vi "Simple Line Detection Control System.vi"() -> ()   [LabVIEW 2017]
panel:
  out "?":string
  in  "Right Sensor":bool=TRUE
  in  "Middle Sensor":bool
  in  "Left Sensor":bool=TRUE
  in  "Stop":bool
  out "Direction":string
  out "Speedometer (m/s)":dbl(knob) scale=0.0..3.0
  in  "% Power":dbl(slide) scale=0.0..100.0
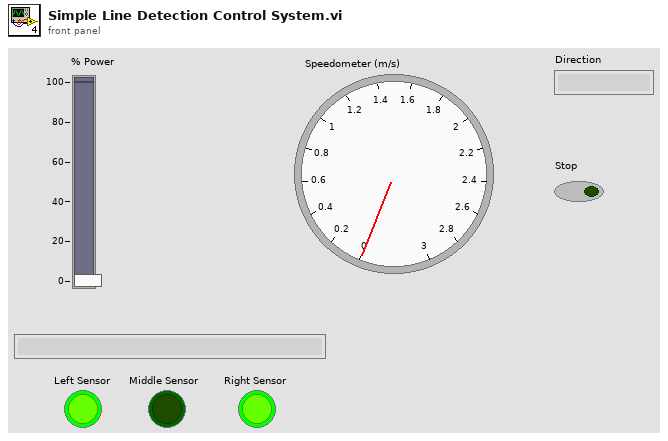
[diagram p1: front panel]
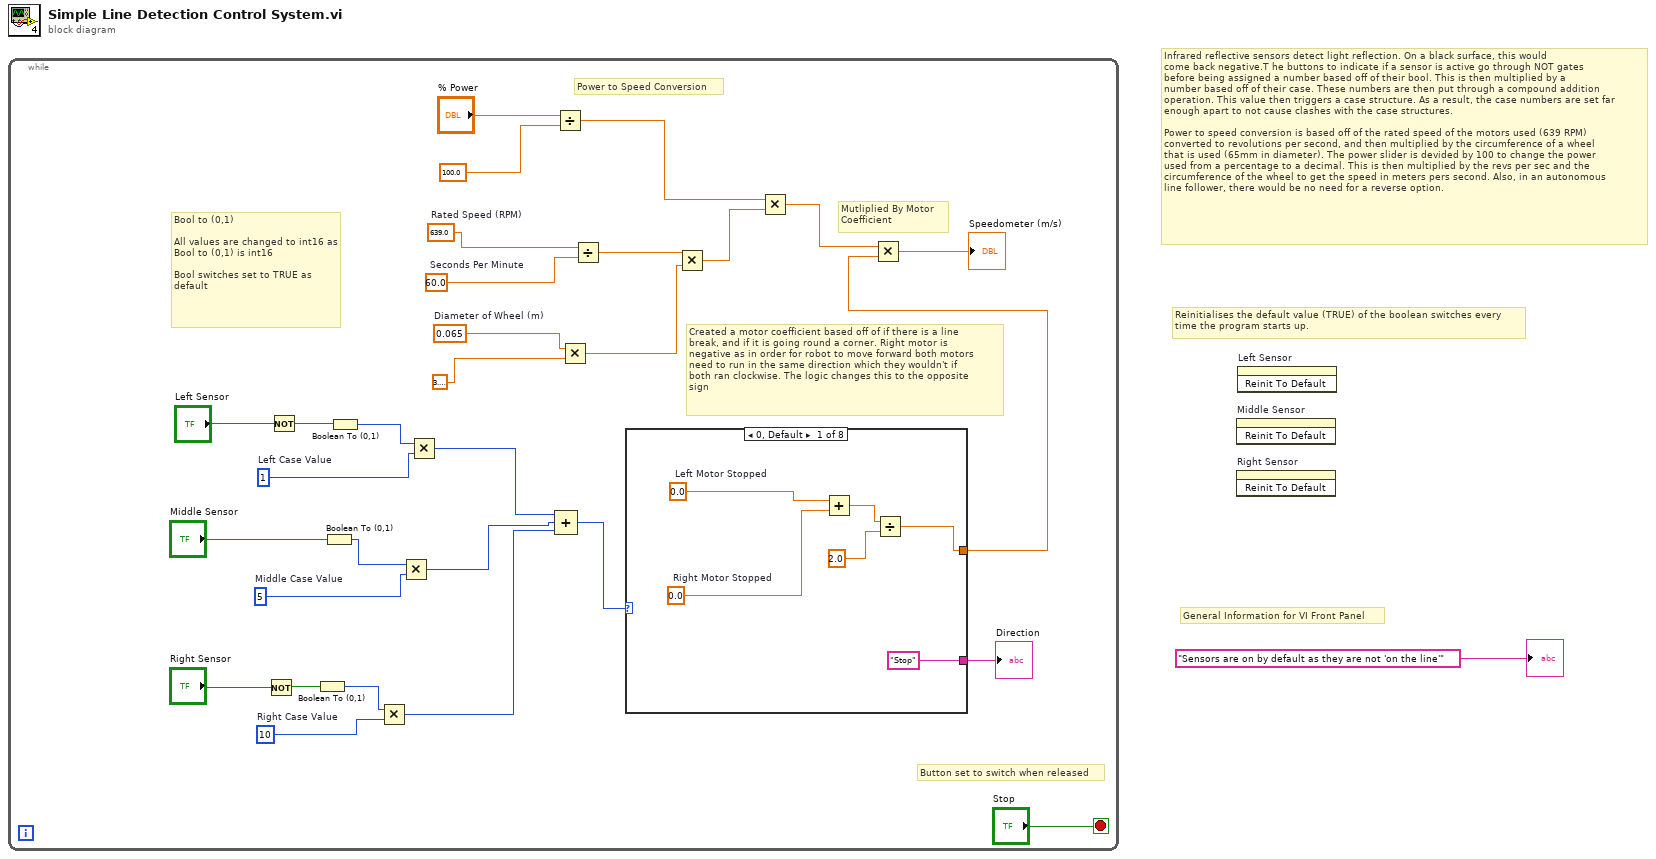
[diagram p0: block diagram]
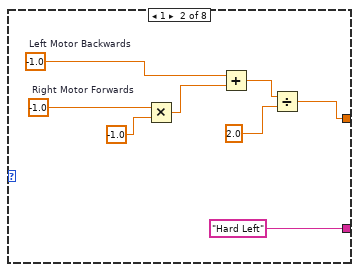
[diagram p2: hidden frame]
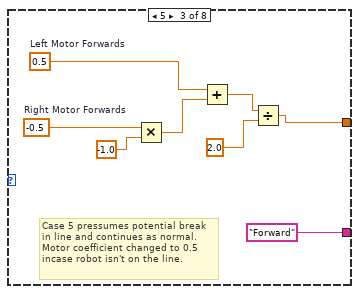
[diagram p3: hidden frame]
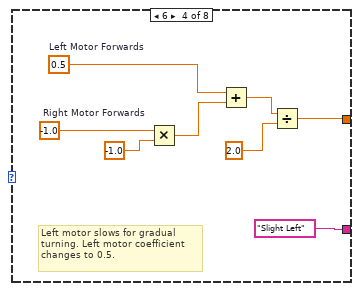
[diagram p4: hidden frame]
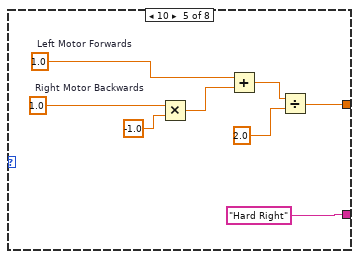
[diagram p5: hidden frame]
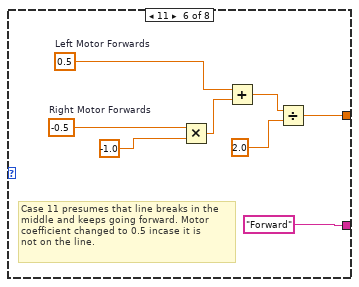
[diagram p6: hidden frame]
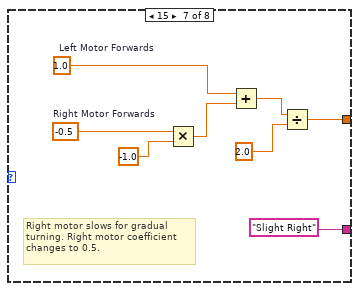
[diagram p7: hidden frame]
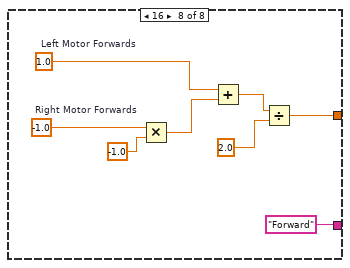
[diagram p8: hidden frame]
diagram:
  # "Reinitialises the default value (TRUE) of the boolean switches every\ntime the program starts up."
  # "General Information for VI Front Panel"
  # "Infrared reflective sensors detect light reflection. On a black surface, this would\ncome back negative.T he buttons to indicate if a sensor is active go through NOT gates\nbefore being assigned a number based off of their bool. This is then multiplied by a \nnumber based off of their case. These numbers are then put through a compound addition\noperation. This value then triggers a case structure. As a result, the case numbers are set far\nenough apart to not cause clashes with the case structures.\n\nPower to speed conversion is based off of the rated speed of the motors used (639 RPM)\nconverted to revolutions per second, and then multiplied by the circumference of a wheel\nthat is used (65mm in diameter). The power slider is devided by 100 to change the power\nused from a percentage to a decimal. This is then multiplied by the revs per sec and the\ncircumference of the wheel to get the speed in meters pers second. Also, in an autonomous\nline follower, there would be no need for a reverse option."
  n1 = while {
    stop <- "Stop" stop-if-true
    w14 = i16 5  # Middle Case Value
    w8 = i16 10  # Right Case Value
    w13 = i16 1  # Left Case Value
    w28 = 0.065  # Diameter of Wheel (m)
    w29 = 60.0  # Seconds Per Minute
    w30 = 639.0  # Rated Speed (RPM)
    # "Created a motor coefficient based off of if there is a line\nbreak, and if it is going round a corner. Right motor is\nnegative as in order for robot to move forward both motors\nneed to run in the same direction which they wouldn't if\nboth ran clockwise. The logic changes this to the opposite\nsign"
    # "Mutliplied By Motor\nCoefficient"
    # "Button set to switch when released"
    # "Bool to (0,1)\n\nAll values are changed to int16 as Bool to (0,1) is int16\n\nBool switches set to TRUE as default"
    # "Power to Speed Conversion"
    n2 = Not(x="Right Sensor") -> (.not. x?=w3:bool)
    n3 = Not(x="Left Sensor") -> (.not. x?=w5:bool)
    n4 = Boolean To (0,1)(Boolean=w3) -> (0, 1=w18:i16)
    n5 = Boolean To (0,1)(Boolean="Middle Sensor") -> (0, 1=w15:i16)
    n6 = Boolean To (0,1)(Boolean=w5) -> (0, 1=w19:i16)
    n7 = Multiply(x=w18, y=w8) -> (x*y=w17:i16)
    n8 = Multiply(x=w15, y=w14) -> (x*y=w16:i16)
    n9 = Multiply(x=w19, y=w13) -> (x*y=w20:i16)
    n10 = Divide(x="% Power", y=100.0) -> (x/y=w21:dbl)
    n11 = Compound Arithmetic op=ADD(w20, w16, w17) -> (w12:i16)
    n12 = Multiply(x=w28, y=3.141592653589793) -> (x*y=w25:dbl)
    n13 = Divide(x=w30, y=w29) -> (x/y=w26:dbl)
    n14 = case shown="0, Default" w12 {
      tunnel: ["Stop" "Hard Left" "Forward" "Slight Left" "Hard Right" "Forward" "Slight Right" "Forward"] -> w31
      tunnel: [w32 w42 w49 w57 w66 w73 w81 w89] -> w7
      frame 0, Default {
        w33 = 0.0  # Right Motor Stopped
        w34 = 0.0  # Left Motor Stopped
        n15 = Add(x=w34, y=w33) -> (x+y=w36:dbl)
        n16 = Divide(x=w36, y=2.0) -> (x/y=w32:dbl)
      }
      frame 1 {
        w39 = -1.0  # Right Motor Forwards
        w41 = -1.0  # Left Motor Backwards
        n17 = Multiply(x=w39, y=-1.0) -> (x*y=w38:dbl)
        n18 = Add(x=w41, y=w38) -> (x+y=w44:dbl)
        n19 = Divide(x=w44, y=2.0) -> (x/y=w42:dbl)
      }
      frame 5 {
        w46 = -0.5  # Right Motor Forwards
        w50 = 0.5  # Left Motor Forwards
        # "Case 5 pressumes potential break\nin line and continues as normal.\nMotor coefficient changed to 0.5\nincase robot isn't on the line."
        n20 = Multiply(x=w46, y=-1.0) -> (x*y=w47:dbl)
        n21 = Add(x=w50, y=w47) -> (x+y=w52:dbl)
        n22 = Divide(x=w52, y=2.0) -> (x/y=w49:dbl)
      }
      frame 6 {
        w55 = -1.0  # Right Motor Forwards
        w58 = 0.5  # Left Motor Forwards
        # "Left motor slows for gradual\nturning. Left motor coefficient\nchanges to 0.5."
        n23 = Multiply(x=w55, y=-1.0) -> (x*y=w54:dbl)
        n24 = Add(x=w58, y=w54) -> (x+y=w60:dbl)
        n25 = Divide(x=w60, y=2.0) -> (x/y=w57:dbl)
      }
      frame 10 {
        w63 = 1.0  # Right Motor Backwards
        w65 = 1.0  # Left Motor Forwards
        n26 = Multiply(x=w63, y=-1.0) -> (x*y=w62:dbl)
        n27 = Add(x=w65, y=w62) -> (x+y=w68:dbl)
        n28 = Divide(x=w68, y=2.0) -> (x/y=w66:dbl)
      }
      frame 11 {
        w71 = -0.5  # Right Motor Forwards
        w74 = 0.5  # Left Motor Forwards
        # "Case 11 presumes that line breaks in the \nmiddle and keeps going forward. Motor\ncoefficient changed to 0.5 incase it is\nnot on the line."
        n29 = Multiply(x=w71, y=-1.0) -> (x*y=w70:dbl)
        n30 = Add(x=w74, y=w70) -> (x+y=w76:dbl)
        n31 = Divide(x=w76, y=2.0) -> (x/y=w73:dbl)
      }
      frame 15 {
        w79 = -0.5  # Right Motor Forwards
        w82 = 1.0  # Left Motor Forwards
        # "Right motor slows for gradual\nturning. Right motor coefficient\nchanges to 0.5."
        n32 = Multiply(x=w79, y=-1.0) -> (x*y=w78:dbl)
        n33 = Add(x=w82, y=w78) -> (x+y=w84:dbl)
        n34 = Divide(x=w84, y=2.0) -> (x/y=w81:dbl)
      }
      frame 16 {
        w86 = -1.0  # Right Motor Forwards
        w90 = 1.0  # Left Motor Forwards
        n35 = Multiply(x=w86, y=-1.0) -> (x*y=w87:dbl)
        n36 = Add(x=w90, y=w87) -> (x+y=w92:dbl)
        n37 = Divide(x=w92, y=2.0) -> (x/y=w89:dbl)
      }
    }
    "Direction" <- w31
    n38 = Multiply(x=w26, y=w25) -> (x*y=w24:dbl)
    n39 = Multiply(x=w21, y=w24) -> (x*y=w9:dbl)
    n40 = Multiply(x=w9, y=w7) -> (x*y=→"Speedometer (m/s)":dbl)
  }
  n41 = invoke on="Middle Sensor" class="Bool (strict)" method="Reinit To Default"() -> ()  [unwired: 3 in, 3 out]
  n42 = invoke on="Right Sensor" class="Bool (strict)" method="Reinit To Default"() -> ()  [unwired: 3 in, 3 out]
  n43 = invoke on="Left Sensor" class="Bool (strict)" method="Reinit To Default"() -> ()  [unwired: 3 in, 3 out]
  "?" <- "Sensors are on by default as they are not 'on the line'"
